vi "MDF4 Set Description.vi"(7 "path in":path, 8 "Error In":errorcluster, 10 "Comment":T1={"Comment"="my comment", "Time Source"="Local PC Reference Time", "Author"="Author", "Department"="Department", "Project"="Project", "Subject"="Subject"}, 11 "MDF4 File Reference in":i64) -> (0 "Error Out":errorcluster, 3 "MDF4 File Reference out":i64)   [LabVIEW 2019, in "MD4Logger Engine.lvlib"]
uses:
  MD4Logger Engine.lvlib
  <vilib>/Utility/error.llb/Error Cluster From Error Code.vi
  <vilib>/ErrorRing/Error Ring.xnode
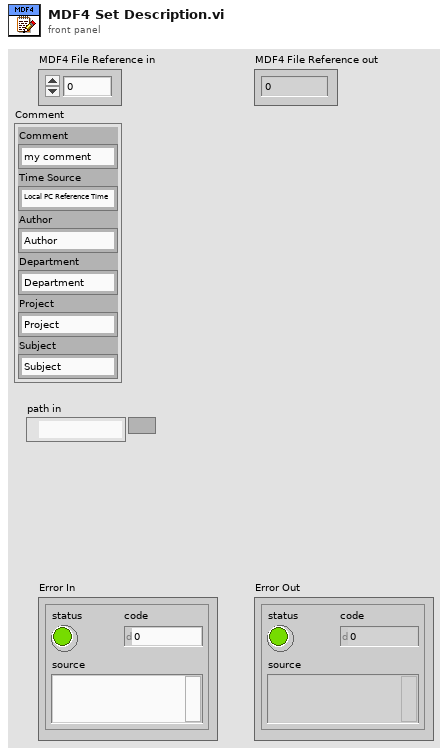
[diagram p1: front panel]
types:
  T1 = cluster{"Comment":string, "Time Source":string, "Author":string, "Department":string, "Project":string, "Subject":string}
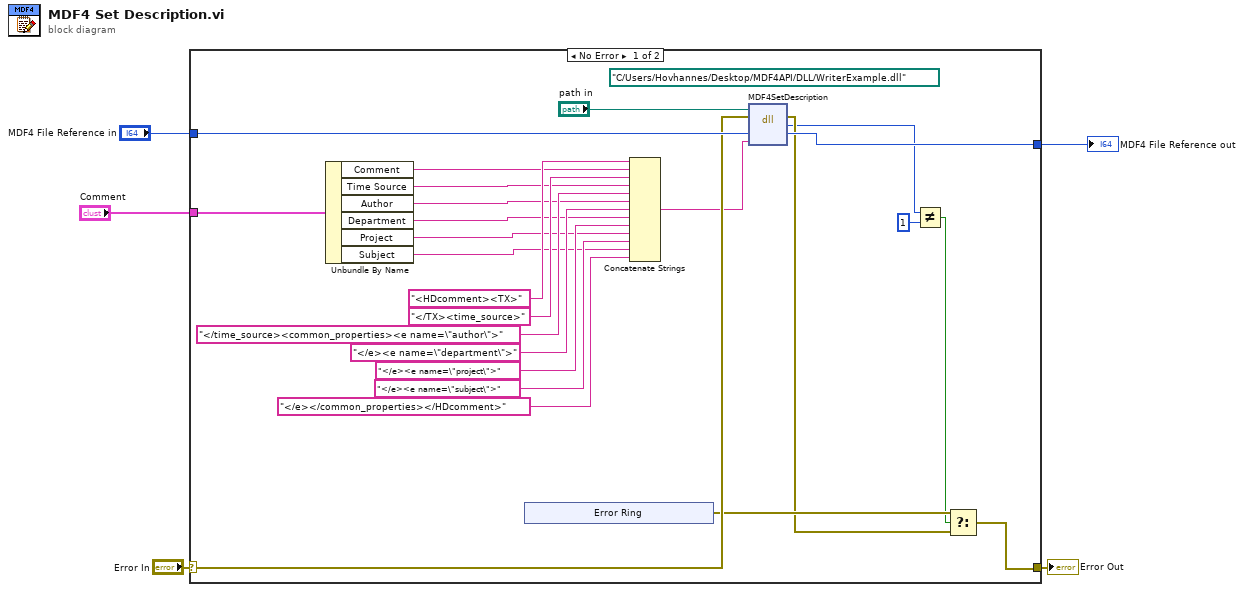
[diagram p0: block diagram]
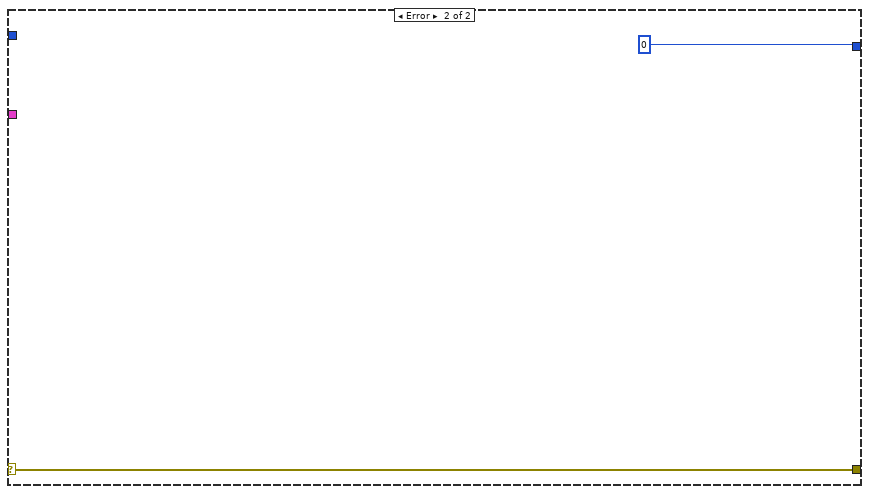
[diagram p2: hidden frame]
diagram:
  n1 = case shown="No Error" "Error In" {
    selector: "Error In" -> [w28 w37]
    tunnel: "MDF4 File Reference in" -> [w30 _]
    tunnel: [w10 w37] -> w3
    tunnel: [w29 i64 0 ("m4")] -> w2
    tunnel: "Comment" -> [w27 _]
    frame No Error {
      (unwired) path "C:/Users/Hovhannes/Desktop/MDF4API/DLL/WriterExample.dll" ("path in")
      n2 = Unbundle By Name(w27) -> ("Comment"=w22:string, "Time Source"=w21:string, "Author"=w20:string, "Department"=w19:string, "Project"=w17:string, "Subject"=w15:string)
      n3 = xnode "Error Ring"() -> ("error out"=w12:errorcluster)
      n4 = Concatenate Strings("<HDcomment><TX>", w22, "</TX><time_source>", w21, "</time_source><common_properties><e name=\"author\">", w20, "</e><e name=\"department\">", w19, "</e><e name=\"project\">", w17, "</e><e name=\"subject\">", w15, "</e></common_properties></HDcomment>") -> (w13:string)
      n5 = dll-call lib="C:/Users/Hovhannes/Desktop/MD4Logger/Source/Engine/DLL/WriterExample.dll" fn="MDF4SetDescription"(path in="path in", error in=w28, "m4"=w30, "description"=w13) -> (error out=w11:errorcluster, "return type"=w7:i32, "m4"=w29:i64)  [unwired: 2 in, 1 out]
      n6 = Not Equal?(x=w7, y=1) -> (x != y?=w8:bool)
      n7 = Select(t=w12, s=w8, f=w11) -> (s? t:f=w10:errorcluster)
    }
    frame Error {
    }
  }
  "MDF4 File Reference out" <- w2
  "Error Out" <- w3
